vi "init_commands.vi"(8 "error in (no error)":errorcluster caption="错误输入（无错误）", 11 "MotorSystem输入":refnum<class "MotorSystem.lvclass">) -> (0 "error out":errorcluster caption="错误输出", 3 "MotorSystem输出":refnum<class "MotorSystem.lvclass">)   [LabVIEW 2016, in "MotionControl.lvlib" / "MotorSystem.lvclass"]
uses:
  <userlib>/MotionControl/MotorSystem/MotorSystem.lvclass
  <userlib>/MotionControl/MotorSystem/cmd_system.ctl
  <userlib>/MotionControl/MotorSystem/MotorSystem.lvclass/MotorSystem.ctl
  <userlib>/MotionControl/OneMotion/OneMotion.lvclass
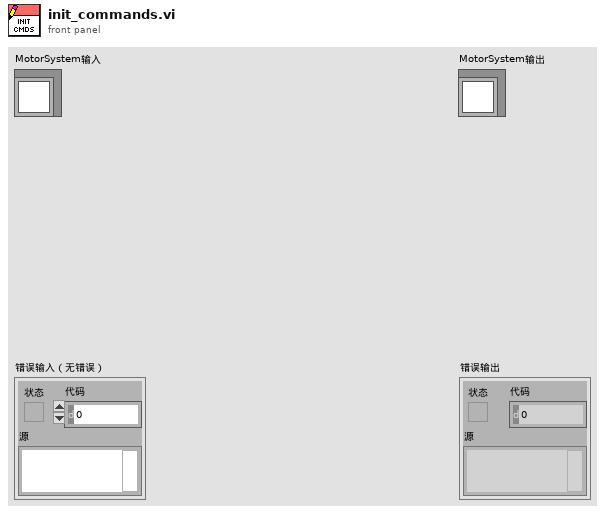
[diagram p1: front panel]
types:
  T1 = typedef "MotionControl.lvlib/MotorSystem.lvclass/cmd_system.ctl" = enum16{"NONE", "MOVE_SYSTEM", "WAIT_UNTIL_MOVE_DONE", "EXIT"}
  T2 = typedef "MotionControl.lvlib/MotorSystem.lvclass/MotionCluster.ctl" = cluster{"OneMotion.lvclass":refnum<class "OneMotion.lvclass">, "connected?":bool, "default enabled?":bool, "enabled?":bool}
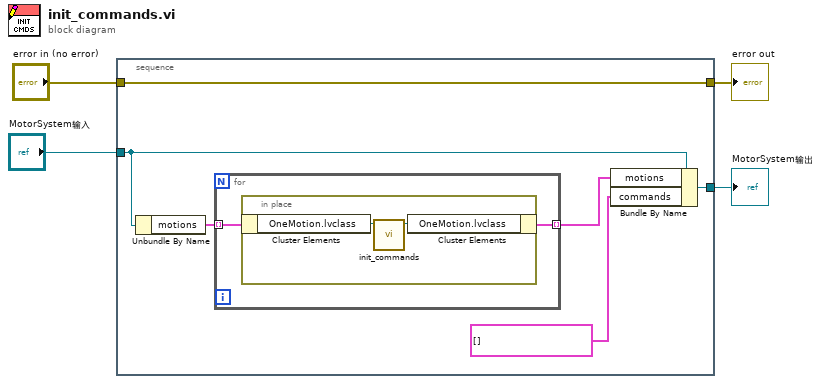
[diagram p0: block diagram]
diagram:
  n1 = stacked-sequence {
    tunnel: [w8] -> w4
    tunnel: [w10] -> w2
    tunnel: "MotorSystem输入" -> [w7]
    tunnel: "error in (no error)" -> [w8]
    frame #0 {
      n2 = Unbundle By Name(w7) -> ("motions"=w6:T2[])
      n3 = for {
        tunnel: w6 -> [w12] mode=indexing
        tunnel: [w11] -> w5 mode=indexing
        n4 = in-place {
          n5 = in-place-cluster #1(w12) -> ("OneMotion.lvclass"=w14:refnum<class "OneMotion.lvclass">)
          n6 = call-dynamic "init_commands.vi"("OneMotion 输入"=w14) -> ("OneMotion 输出"=w13:refnum<class "OneMotion.lvclass">)  [unwired: 9 in, 1 out]
          n7 = in-place-cluster #1("OneMotion.lvclass"=w13) -> (w11:T2)
        }
      }
      n8 = Bundle By Name(cluster=w7, "motions"=w5, "commands"=cluster{"cmd":T1, "cmd data":variant}[] []) -> (w10:refnum<class "MotorSystem.lvclass">)
    }
  }
  "error out" <- w4
  "MotorSystem输出" <- w2
